vi "UTILITY Common PID Adjuster.vi"(0 "Previous Value":dbl, 1 "Current Rate":dbl, 2 "Scan Rate Target":dbl, 3 "K(7) - Adjustment Factor":dbl, 4 "ErrorPassBand(%)":dbl, 5 "Error In":errorcluster, 6 "Use Fuzzy Logic":bool, 7 "Use Proportion Valve":bool, 8 "PID gains":T1={"proportional gain (Kc)"=0.1, "integral time (Ti, min)"=0.01, "derivative time (Td, min)"=0.0} {"derivative time (Td, min)" format="%.3f"; "integral time (Ti, min)" format="%.3f"; "proportional gain (Kc)" format="%.3f"}, 10 "output range":cluster{"output high":dbl, "output low":dbl}={"output high"=140.0, "output low"=40.0} {"output low" format="%.2f"; "output high" format="%.2f"}) -> (14 "New MicroAmp":dbl, 15 "Going into Correction Loop?":bool, 16 "Adjustment Factor":dbl, 19 "Error Out":errorcluster)   [LabVIEW 2016]
uses:
  <vilib>/addons/control/pid/pid.llb/PID (DBL).vi
  <vilib>/addons/control/pid/NI_PID_pid.lvlib
panel:
  out "dt out (s)":dbl format="%.3f"
  in  "reinitialize? (F)":bool
  in  "dt (s)":dbl=0.5 format="%#_13g"
  out "Fuzzy Logic Temp":dbl=60.005300916477566 format="%.2f"
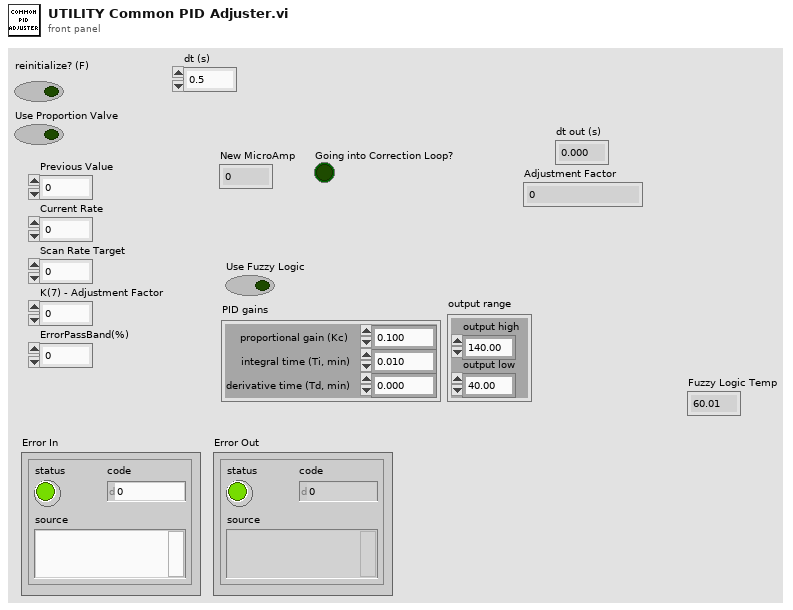
[diagram p1: front panel]
types:
  T1 = cluster{"proportional gain (Kc)":dbl, "integral time (Ti, min)":dbl, "derivative time (Td, min)":dbl}
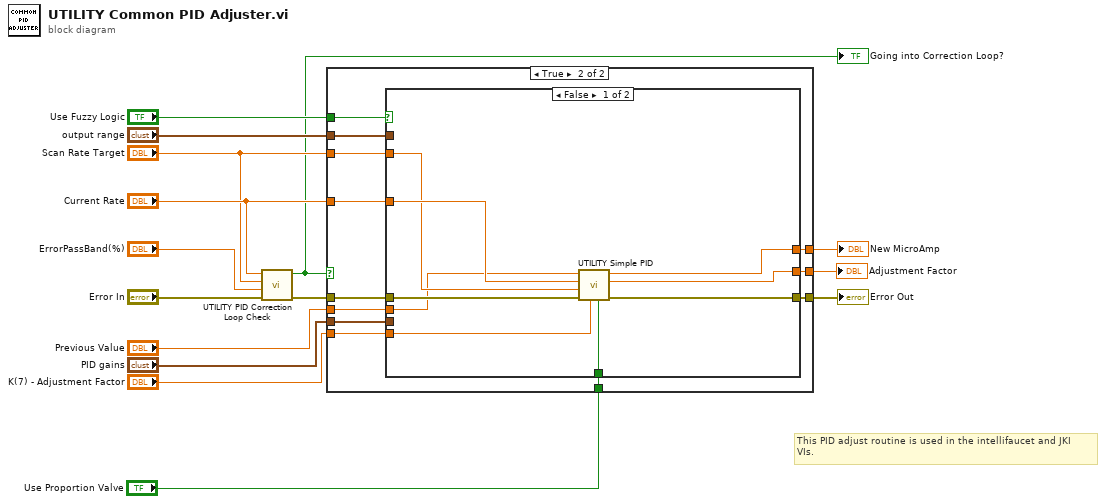
[diagram p0: block diagram]
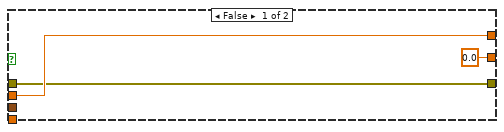
[diagram p2: hidden frame]
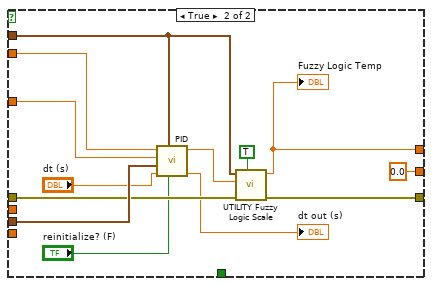
[diagram p3: hidden frame]
diagram:
  # "This PID adjust routine is used in the intellifaucet and JKI \nVIs."
  n1 = call "UTILITY PID Correction Loop Check.vi"("Error In"="Error In", "ErrorPassBand(%)"="ErrorPassBand(%)", "GPM Target(3)"="Scan Rate Target", "GPM reading"="Current Rate") -> ("Error Out"=w13:errorcluster, "Going into Correction Loop?"=w3:bool)  [unwired: 6 in]
  "Going into Correction Loop?" <- w3
  n2 = case shown="True" w3 {
    tunnel: w13 -> [w17 w30]
    tunnel: "Current Rate" -> [_ w29]
    tunnel: "Scan Rate Target" -> [_ w28]
    tunnel: [w18 w27] -> w9
    tunnel: "Previous Value" -> [w18 w26]
    tunnel: "K(7) - Adjustment Factor" -> [_ w25]
    tunnel: "PID gains" -> [_ w24]
    tunnel: "output range" -> [_ w23]
    tunnel: "Use Fuzzy Logic" -> [_ w22]
    tunnel: [w17 w21] -> w4
    tunnel: [0.0 ("Adjustment Factor") w20] -> w2
    tunnel: "Use Proportion Valve" -> [_ w19]
    frame False {
    }
    frame True {
      n3 = case shown="False" w22 {
        tunnel: w30 -> [w39 w44]
        tunnel: w29 -> [w38 w43]
        tunnel: w28 -> [w37 w52]
        tunnel: [w36 w47] -> w27
        tunnel: w26 -> [w35 _]
        tunnel: w25 -> [w34 _]
        tunnel: w24 -> [_ w51]
        tunnel: w23 -> [_ w45]
        tunnel: [w33 w49] -> w21
        tunnel: [w32 0.0 ("Adjustment Factor")] -> w20
        tunnel: w19 -> [w31 _]
        frame False {
          n4 = call "UTILITY Simple PID.vi"("Use Proportion Valve"=w31, "K(0.1)"=w34, "Error In"=w39, "GPM Target(3)"=w37, "GPM reading"=w38, "Previous MicroAmp"=w35) -> ("Error Out"=w33:errorcluster, "Adjustment Factor"=w32:dbl, "New MicroAmp"=w36:dbl)  [unwired: 3 in]
        }
        frame True {
          n5 = call-poly <vilib>:"PID.vi"("reinitialize? (F)"="reinitialize? (F)", "output range"=w45, "dt (s)"="dt (s)", "PID gains"=w51, "process variable"=w43, "setpoint"=w52) -> ("dt out (s)"=→"dt out (s)":dbl, "output"=w48:dbl)  [unwired: 4 in]
          n6 = call "UTILITY Fuzzy Logic Scale.vi"("Convert to MicroAmp (T), Standard Output (F)"=TRUE, "Error In"=w44, "input variable"=w48, "output range"=w45) -> ("Error Out"=w49:errorcluster, "MicroAmp"=w47:dbl)  [unwired: 6 in]
          "Fuzzy Logic Temp" <- w47
        }
      }
    }
  }
  "New MicroAmp" <- w9
  "Error Out" <- w4
  "Adjustment Factor" <- w2
